vi "InitScrollbarAndListBox.vi"(5 "control refs":T2, 7 "configuration":T3, 8 "error in (no error)":errorcluster, 9 "channel names":string[](array[string]), 10 "group names":string[](array[string]), 11 "TDMS descriptor array":T1(array[cluster])) -> (0 "error out":errorcluster, 1 "channel out":string[](array[string]), 2 "group out":string[](array[string]), 3 "TDMS descriptor array out":T1(array[cluster]))   [LabVIEW 2015]
uses:
  <vilib>/Utility/tdmsutil.llb/fileViewerConfigData.ctl
panel:
  out "tdms out":refnum<k34>
  in  "tdms in":refnum<k34>
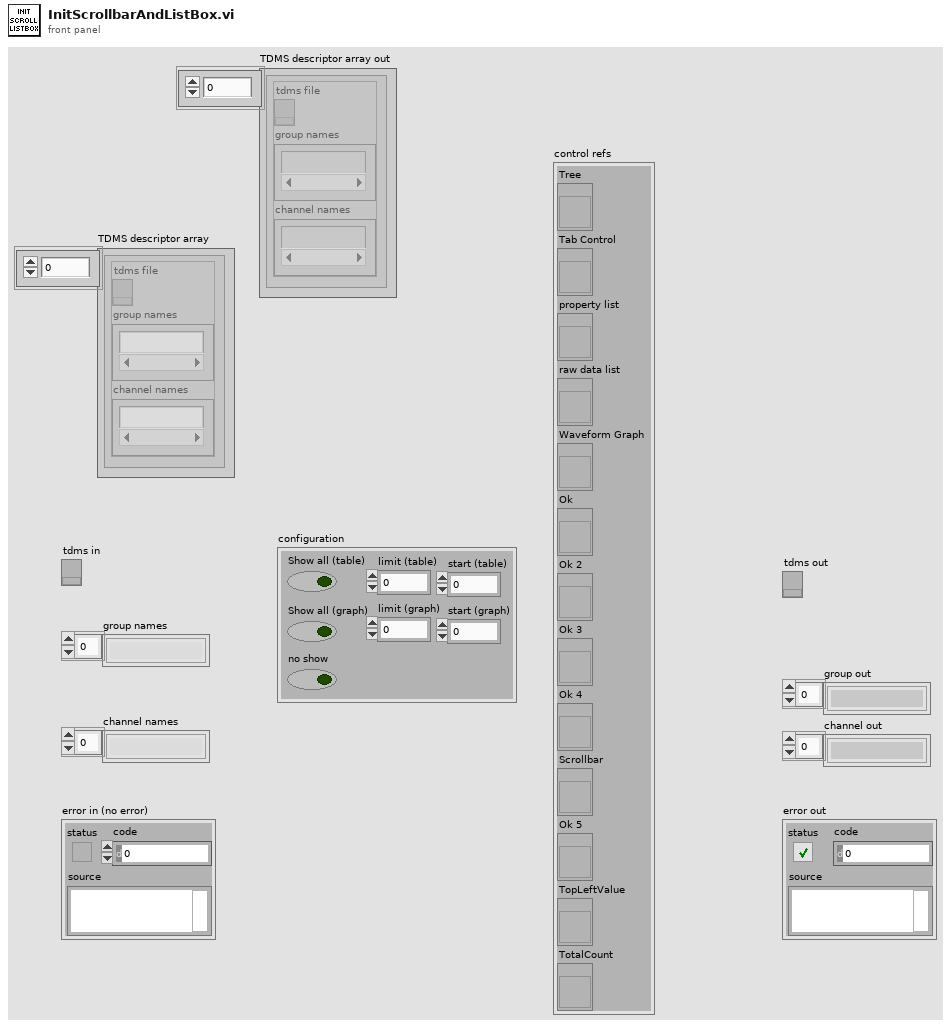
[diagram p1: front panel]
types:
  T1 = cluster{"tdms file ":refnum<k34>, "group names":string[], "channel names":string[]}[]
  T2 = cluster{"Tree":refnum<vi>, "Tab Control":refnum<vi>, "property list":refnum<vi>, "raw data list":refnum<vi>, "Waveform Graph":refnum<vi>, "Ok":refnum<vi>, "Ok 2":refnum<vi>, "Ok 3":refnum<vi>, "Ok 4":refnum<vi>, "Scrollbar":refnum<vi>, "Ok 5":refnum<vi>, "TopLeftValue":refnum<vi>, "TotalCount":refnum<vi>}
  T3 = typedef "fileViewerConfigData.ctl" = cluster{"Show all (table)":bool, "Show all (graph)":bool, "limit (table)":u64, "limit (graph)":u64, "no show":bool, "start (table)":u64, "start (graph)":u64}
  T4 = cluster{"tdms file ":refnum<k34>, "group names":string[], "channel names":string[]}
  T5 = typedef "LVRowAndColumnUnsignedTypeDef.ctl" = cluster{"Row":u32, "Column":u32}
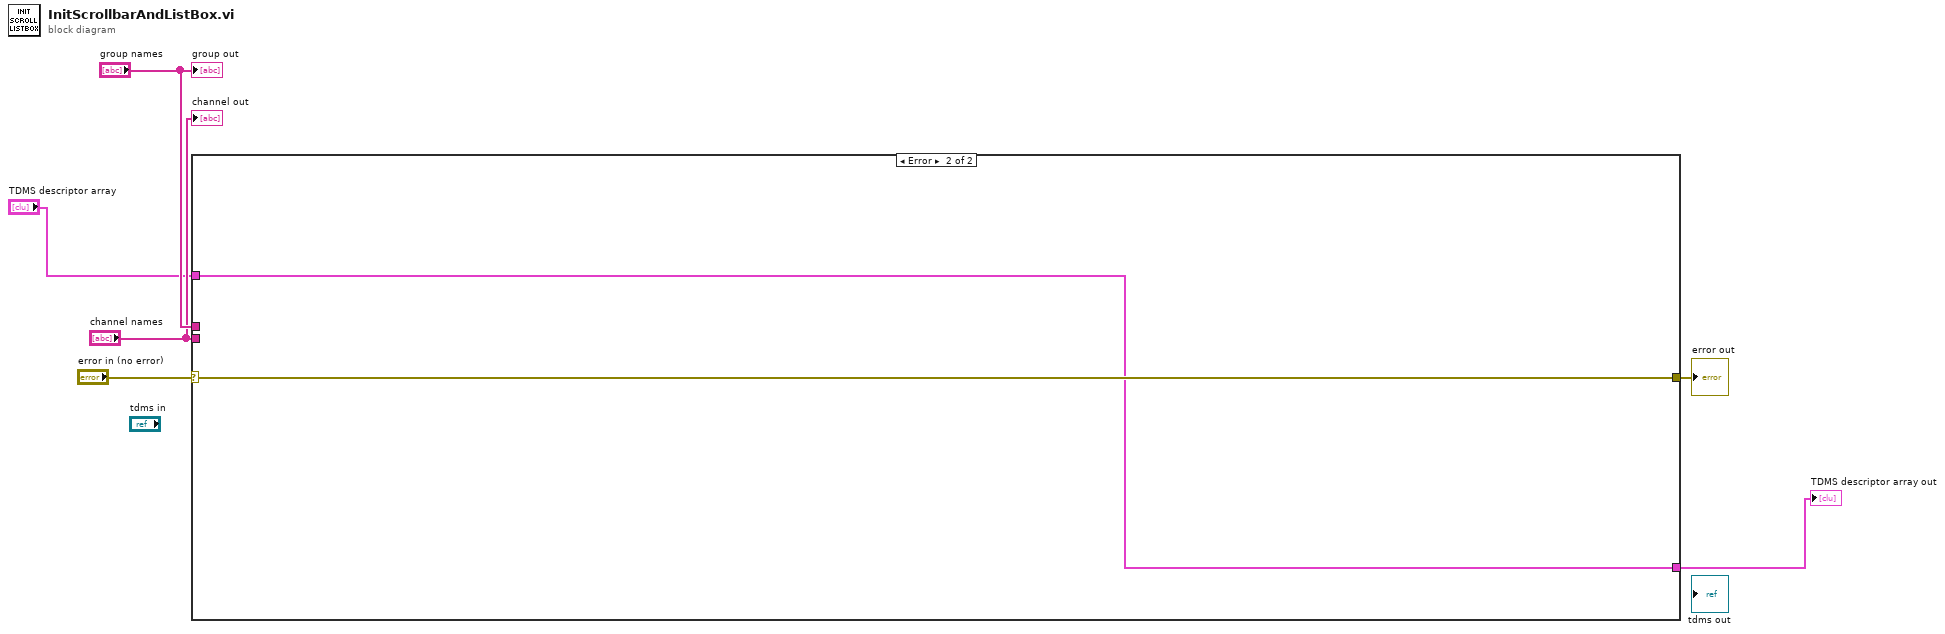
[diagram p0: block diagram]
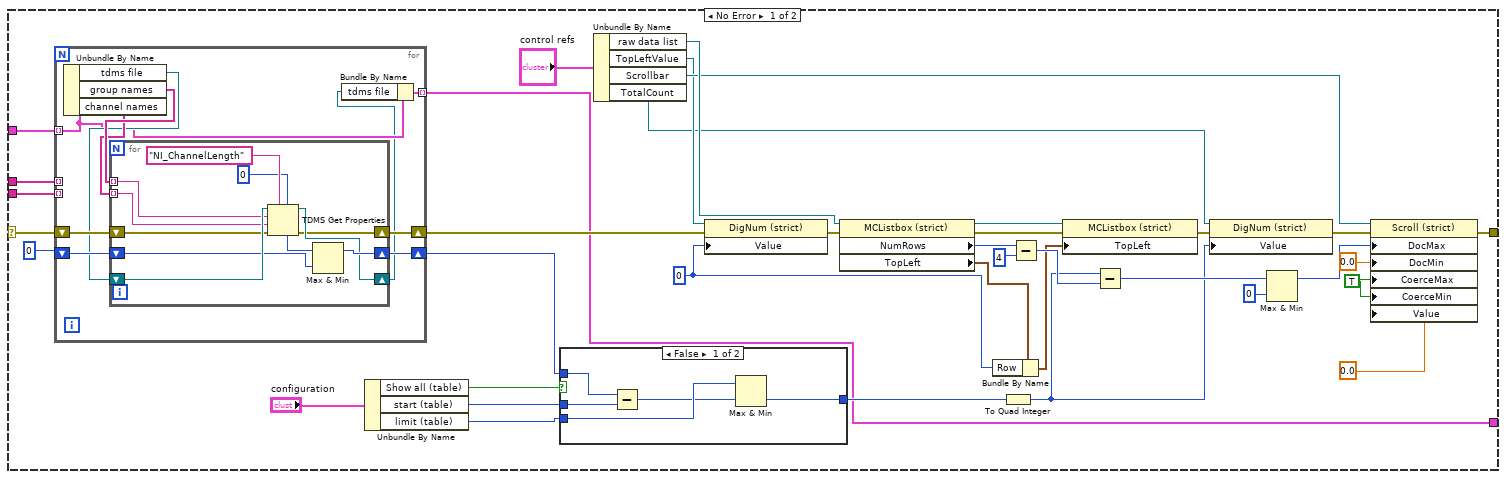
[diagram p2: hidden frame]
diagram:
  n1 = case shown="Error" "error in (no error)" {
    selector: "error in (no error)" -> [w15 w72]
    tunnel: "group names" -> [w39 _]
    tunnel: "channel names" -> [w37 _]
    tunnel: [w16 w72] -> w4
    tunnel: "TDMS descriptor array" -> [w9 w71]
    tunnel: [w7 w71] -> w1
    frame No Error {
      w24 = u64 0 ("LastLeftTopRow")
      w36 = TRUE ("Coerce Maximum Value")
      n2 = for {
        tunnel: w39 -> [_] mode=indexing
        tunnel: w37 -> [_] mode=indexing
        shift-right: [w52] -> w19
        shift-left: w15 -> [w51]
        tunnel: w9 -> [w46] mode=indexing
        shift-right: [w53] -> w42
        shift-left: u64 0 -> [w48]
        tunnel: [w44] -> w7 mode=indexing
        n3 = Unbundle By Name(w46) -> ("tdms file"=w47:refnum<k34>, "group names"=w50:string[], "channel names"=w49:string[])
        n4 = for {
          tunnel: w50 -> [w63] mode=indexing
          tunnel: w49 -> [w62] mode=indexing
          shift-right: [w56] -> w53
          shift-left: w48 -> [w57]
          shift-right: [w54] -> w52
          shift-left: w51 -> [w61]
          shift-right: [w55] -> w45
          shift-left: w47 -> [w64]
          n5 = TDMS Get Properties(5:u64 0, 7:"NI_ChannelLength" ("property name"), 8:w61, 9:w62, 10:w63, 11:w64) -> (0:w54:errorcluster, 3:w55:refnum<k34>, 4:w58:u64)  [unwired: 3 out]
          n6 = Max & Min(x=w58, y=w57) -> (max(x,y)=w56:u64)  [unwired: 1 out]
        }
        n7 = Bundle By Name(cluster=w46, "tdms file"=w45) -> (w44:T4)
      }
      n8 = Unbundle By Name("configuration") -> ("Show all (table)"=w43:bool, "start (table)"=w40:u64, "limit (table)"=w41:u64)
      n9 = case shown="False" w43 {
        tunnel: w42 -> [w68 w70]
        tunnel: w41 -> [w69 _]
        tunnel: w40 -> [w67 _]
        tunnel: [w65 w70] -> w21
        frame False {
          n10 = Subtract(x=w68, y=w67) -> (x-y=w66:u64)
          n11 = Max & Min(x=w69, y=w66) -> (min(x,y)=w65:u64)  [unwired: 1 out]
        }
        frame True {
        }
      }
      n12 = Unbundle By Name("control refs") -> ("raw data list"=w27:refnum<vi>, "TopLeftValue"=w25:refnum<vi>, "Scrollbar"=w26:refnum<vi>, "TotalCount"=w13:refnum<vi>)
      n13 = property class="DigNum (strict)"(reference=w25, error in=w19, "Value"=w24) -> (error out=w18:errorcluster)  [unwired: 1 out]
      n14 = property on="Property Node" class="MCListbox (strict)"(reference=w27, error in=w18) -> (reference out=w20:refnum<vi>, error out=w17:errorcluster, "NumRows"=w30:u32, "TopLeft"=w23:T5)
      n15 = Bundle By Name(cluster=w23, "Row"=w24) -> (w22:T5)
      n16 = To Quad Integer(1:w21) -> (0:w10:i64)
      n17 = Subtract(x=w30, y=u32 4) -> (x-y=w28:u32)
      n18 = property on="Property Node" class="MCListbox (strict)"(reference=w20, error in=w17, "TopLeft"=w22) -> (error out=w12:errorcluster)  [unwired: 1 out]
      n19 = Subtract(x=w10, y=w28) -> (x-y=w33:i64)
      n20 = property class="DigNum (strict)"(reference=w13, error in=w12, "Value"=w10) -> (error out=w11:errorcluster)  [unwired: 1 out]
      n21 = Max & Min(x=w33, y=i64 0) -> (max(x,y)=w31:i64)  [unwired: 1 out]
      n22 = property on="Property Node" class="Scroll (strict)"(reference=w26, error in=w11, "DocMax"=w31, "DocMin"=0.0 ("Doc Min"), "CoerceMax"=w36, "CoerceMin"=w36, "Value"=0.0 ("Scrollbar")) -> (error out=w16:errorcluster)  [unwired: 1 out]
    }
    frame Error {
    }
  }
  "error out" <- w4
  "TDMS descriptor array out" <- w1
  "group out" <- "group names"
  "channel out" <- "channel names"
